vi "Initialize General Settings Tree.vi"(11 "UI Data in":refnum<class "Settings UI.lvclass">) -> (2 "Items to Add":T1(array[cluster]), 3 "UI Data out":refnum<class "Settings UI.lvclass">)   [LabVIEW 2020, in "Output Sequencer.lvlib" / "Settings UI.lvclass"]
uses:
  Settings UI.lvclass
  Types/Tree Index Enum.ctl
  Settings UI.lvclass/Settings UI.ctl
  Globals/Global Tree Data.vi
  Output Sequencer/Globals/Global Strings.vi
  Output Sequencer/Output Sequencer.lvclass
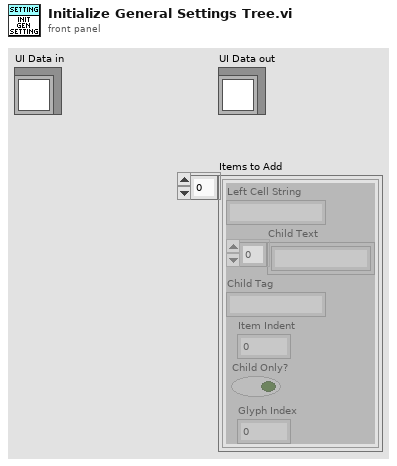
[diagram p1: front panel]
types:
  T1 = cluster{"Left Cell String":string, "Child Text":string[], "Child Tag":string, "Item Indent":i32, "Child Only?":bool, "Glyph Index":i32}[]
  T2 = typedef "Output Sequencer.lvlib/Settings UI.lvclass/Tree Index Enum.ctl" = enum16{"General Settings", "Num Steps", "Num Analog", "Num Digital", "Show Confirmation", "Interp Priority", "Adv Timing", "Enable Conditions", "Seq Execution", "Reset Test Start", "Only When Test", "Delay After Test", "Start condition", "Re-triggering", "Stop condition", "Stop After Cycles", "Stop Values", "Default Values", "Default Analog", "Default Digital", "Steps", "Step #", "Description", "Precondition", "Duration", "Mode", "Delay Between Vals", "Analog Values", "Digital Values", "Postcondition", "On True", "On False"}
  T3 = typedef "Output Sequencer.lvlib/Settings UI.lvclass/Tree Item Settings.ctl" = cluster{"Tree Label":string, "Indent Level":i32, "Data Type":T4, "Numeric Range":cluster{"Min":dbl, "Max":dbl, "Inc":dbl}, "Allowed Values":string[], "Default Value":string, "Description":string}
  T4 = typedef "Output Sequencer.lvlib/Settings UI.lvclass/Data Type.ctl" = i16
  T5 = cluster{"Left Cell String":string, "Child Text":string[], "Child Tag":string, "Item Indent":i32, "Child Only?":bool, "Glyph Index":i32}
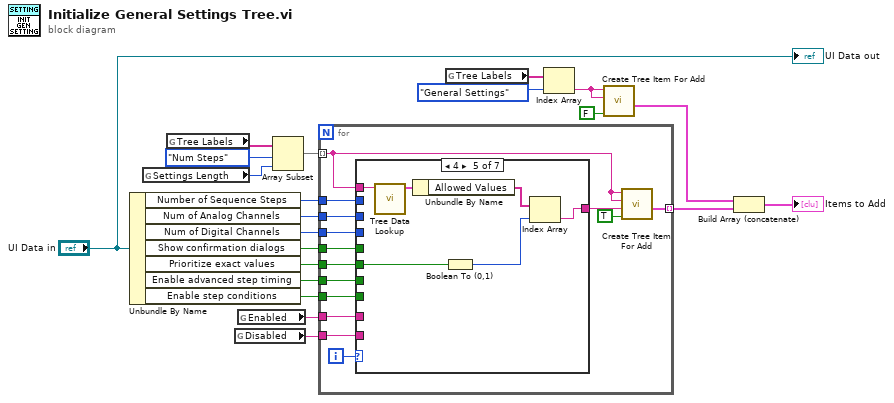
[diagram p0: block diagram]
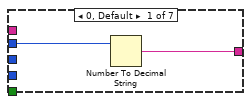
[diagram p2: hidden frame]
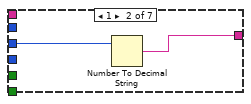
[diagram p3: hidden frame]
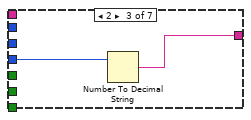
[diagram p4: hidden frame]
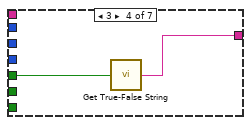
[diagram p5: hidden frame]
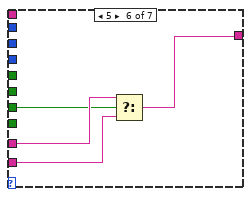
[diagram p6: hidden frame]
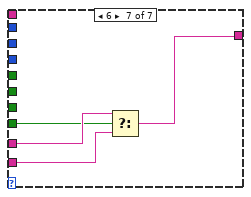
[diagram p7: hidden frame]
diagram:
  n1 = Unbundle By Name("UI Data in") -> ("Number of Sequence Steps"=w3:i32, "Num of Analog Channels"=w4:i32, "Num of Digital Channels"=w5:i32, "Show confirmation dialogs"=w19:bool, "Prioritize exact values"=w18:bool, "Enable advanced step timing"=w12:bool, "Enable step conditions"=w13:bool)
  n2 = global read "Global Tree Data.vi" "Settings Length"() -> (w8:i32)
  n3 = global read "Global Tree Data.vi" "Tree Labels"() -> (w6:string[])
  n4 = global read "Global Strings.vi" "Disabled"() -> (w17:string)
  n5 = global read "Global Strings.vi" "Enabled"() -> (w16:string)
  n6 = Array Subset(array=w6, index=Tree_Index_Enum."Num Steps" ("Tree Index Enum"), length=w8) -> (w7:string[])
  n7 = for {
    tunnel: w7 -> [w27] mode=indexing
    tunnel: w3 -> [w35]
    tunnel: w4 -> [w34]
    tunnel: w5 -> [w33]
    tunnel: [w31] -> w1 mode=indexing
    tunnel: w18 -> [w28]
    tunnel: w12 -> [w26]
    tunnel: w13 -> [w25]
    tunnel: w16 -> [w24]
    tunnel: w17 -> [w23]
    tunnel: w19 -> [w22]
    i -> [w32]
    n8 = case shown="4" w32 {
      tunnel: w35 -> [w37 _ _ _ _ _ _]
      tunnel: w34 -> [_ w39 _ _ _ _ _]
      tunnel: w33 -> [_ _ w41 _ _ _ _]
      tunnel: [w36 w38 w40 w42 w45 w50 w55] -> w30
      tunnel: w28 -> [_ _ _ _ w44 _ _]
      tunnel: w27 -> [_ _ _ _ w49 _ _]
      tunnel: w26 -> [_ _ _ _ _ w51 _]
      tunnel: w25 -> [_ _ _ _ _ _ w54]
      tunnel: w24 -> [_ _ _ _ _ w53 w57]
      tunnel: w23 -> [_ _ _ _ _ w52 w56]
      tunnel: w22 -> [_ _ _ w43 _ _ _]
      frame 0, Default {
        n9 = Number To Decimal String(number=w37) -> (decimal integer string=w36:string)  [unwired: 1 in]
      }
      frame 1 {
        n10 = Number To Decimal String(number=w39) -> (decimal integer string=w38:string)  [unwired: 1 in]
      }
      frame 2 {
        n11 = Number To Decimal String(number=w41) -> (decimal integer string=w40:string)  [unwired: 1 in]
      }
      frame 3 {
        n12 = call "Get True-False String.vi"("Input"=w43) -> ("True/False String"=w42:string)
      }
      frame 4 {
        n13 = call "Tree Data Lookup.vi"("Tag in"=w49) -> ("Tree Data"=w48:T3)  [unwired: 5 in, 5 out]
        n14 = Unbundle By Name(w48) -> ("Allowed Values"=w47:string[])
        n15 = Boolean To (0,1)(Boolean=w44) -> (0, 1=w46:i16)
        n16 = Index Array(array=w47, index=w46) -> (element=w45:string)
      }
      frame 5 {
        n17 = Select(t=w53, s=w51, f=w52) -> (s? t:f=w50:string)
      }
      frame 6 {
        n18 = Select(t=w57, s=w54, f=w56) -> (s? t:f=w55:string)
      }
    }
    n19 = call "Create Tree Item For Add.vi"("Child Only? (true)"=TRUE ("Child Only? (False)"), "Child Text"=w30, "Left Cell String"=w27, "Child Tag in"=w27) -> ("Item"=w31:T5)  [unwired: 6 in, 1 out]
  }
  n20 = global read "Global Tree Data.vi" "Tree Labels"() -> (w9:string[])
  n21 = Index Array(array=w9, index=Tree_Index_Enum."General Settings" ("Tree Index Enum")) -> (element=w10:string)
  n22 = call "Create Tree Item For Add.vi"("Child Only? (true)"=FALSE, "Left Cell String"=w10, "Child Tag in"=w10) -> ("Item"=w2:T5)  [unwired: 7 in, 1 out]
  n23 = Build Array (concatenate)(w2, w1) -> (→"Items to Add":T1)
  "UI Data out" <- "UI Data in"
